vi "exec.vi"(8 "error in (no error)":errorcluster, 10 "context":refnum<class "IContextThisComponent.lvclass">, 11 "CaptureSpectImage in":refnum<class "captureSpectImage.lvclass">) -> (0 "error out":errorcluster, 2 "context 2":refnum<class "IContextThisComponent.lvclass">, 3 "CaptureSpectImage out":refnum<class "captureSpectImage.lvclass">)   [LabVIEW 2016, in "Commands.lvlib" / "captureSpectImage.lvclass"]
uses:
  captureSpectImage.lvclass
  IContextThisComponent/IContextThisComponent.lvclass
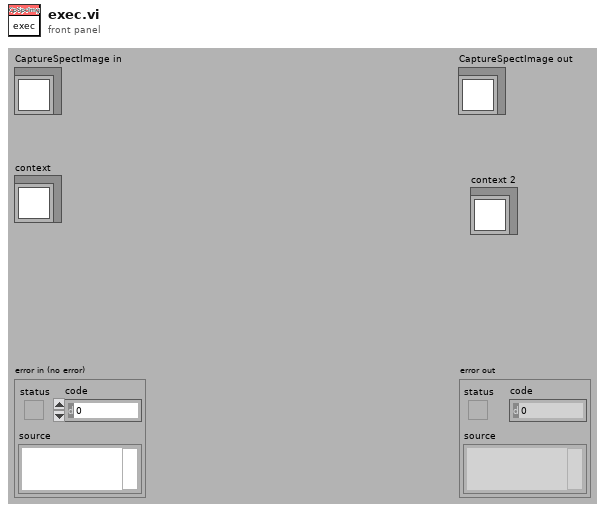
[diagram p1: front panel]
types:
  T1 = typedef "SALLV_sedSpectrometer.lvlib/command_captureSpectImage.ctl" = cluster{"integrationTime":sgl, "imageType":string, "lamp":string}
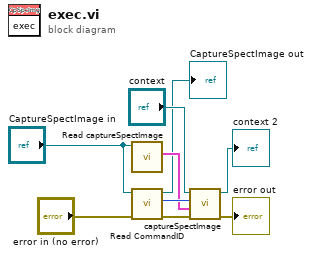
[diagram p0: block diagram]
diagram:
  n1 = call-dynamic "Read captureSpectImage.vi"("captureSpectImage in"="CaptureSpectImage in") -> ("command_captureSpectImage"=w2:T1)  [unwired: 8 in, 2 out]
  n2 = call-dynamic "Read CommandID.vi"("error in (no error)"="error in (no error)", "Command in"="CaptureSpectImage in") -> ("error out"=w4:errorcluster, "CommandID"=w8:i32, "Command out"=→"CaptureSpectImage out":refnum<class "captureSpectImage.lvclass">)  [unwired: 7 in]
  n3 = call-dynamic "captureSpectImage.vi"("error in (no error)"=w4, "captureSpectImage"=w2, "CommandID"=w8, "IContextThisComponent in"="context") -> ("error out"=→"error out":errorcluster, "IContextThisComponent out"=→"context 2":refnum<class "IContextThisComponent.lvclass">)  [unwired: 5 in]
